vi "Get RTD Type.vi"(8 "error in (no error)":errorcluster, 11 "VISA resource name":refnum<visa-resource-name>) -> (0 "error out":errorcluster, 2 "RTD Sensor":i32, 3 "VISA resource name out":refnum<visa-resource-name>)   [LabVIEW 2013, in "Fluke 5XXX Series Multicalibrators.lvlib"]
doc: "This VI returns the Resistance Temperature Detector (RTD) type used for RTD temperature simulations.\n\nNote:\n\nThis VI is available only for instrument models 5500A and 5520A."
uses:
  Fluke 5XXX Series Multicalibrators.lvlib
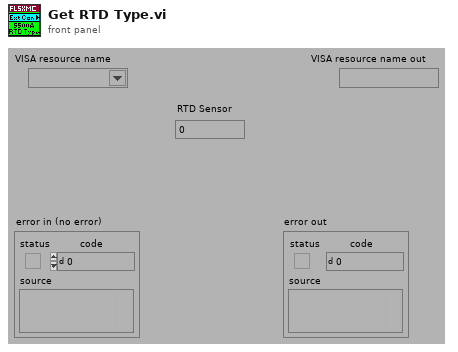
[diagram p1: front panel]
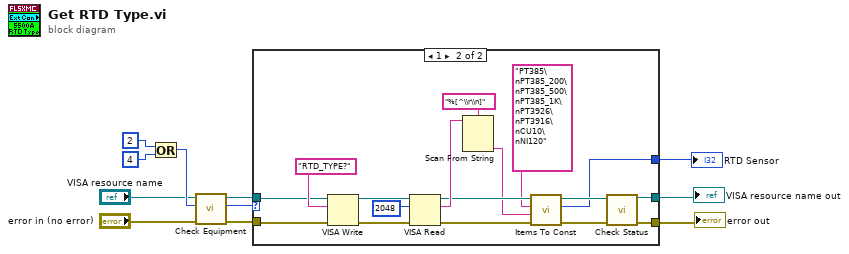
[diagram p0: block diagram]
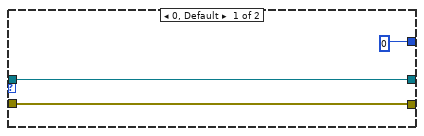
[diagram p2: hidden frame]
diagram:
  n1 = Or(x=2 ("Numeric"), y=4 ("Numeric")) -> (x .or. y?=w6:i32)
  n2 = call "Check Equipment.vi"("error in (no error)"="error in (no error)", "Bit Mask"=w6, "VISA resource name"="VISA resource name") -> ("error out"=w11:errorcluster, "Present?"=w10:u32, "VISA resource name out"=w9:refnum<visa-resource-name>)  [unwired: 6 in]
  n3 = case shown="1" w10 {
    tunnel: [w14 w25] -> w3
    tunnel: [w13 w24] -> w2
    tunnel: w11 -> [w14 w27]
    tunnel: w9 -> [w13 w26]
    tunnel: [0 w17] -> w1
    frame 0, Default {
    }
    frame 1 {
      n4 = VISA Write(VISA resource name=w26, write buffer="RTD_TYPE?", error in (no error)=w27) -> (VISA resource name out=w30:refnum<visa-resource-name>, error out=w29:errorcluster)  [unwired: 1 out]
      n5 = VISA Read(VISA resource name=w30, byte count=u32 2048 ("byte count (0)"), error in (no error)=w29) -> (VISA resource name out=w19:refnum<visa-resource-name>, read buffer=w22:string, error out=w20:errorcluster)  [unwired: 1 out]
      n6 = Scan From String(format string="%[^\\r\\n]", input string=w22) -> (output 1=w15:string)  [unwired: 3 in, 3 out]
      n7 = call "Items To Const.vi"("error in (no error)"=w20, "String Item"=w15, "Multi-Line String"="PT385\nPT385_200\nPT385_500\nPT385_1K\nPT3926\nPT3916\nCU10\nNI120", "VISA resource name"=w19) -> ("error out"=w21:errorcluster, "Index"=w17:i32, "VISA resource name out"=w18:refnum<visa-resource-name>)  [unwired: 5 in]
      n8 = call "Check Status.vi"("VISA resource name"=w18, "error in (no error)"=w21) -> ("VISA resource name out"=w24:refnum<visa-resource-name>, "error out"=w25:errorcluster)  [unwired: 12 in]
    }
  }
  "RTD Sensor" <- w1
  "VISA resource name out" <- w2
  "error out" <- w3
